vi "RP-GEN SINUS-OUT.vi"(1 "Amplitude(1V)":dbl=1.0, 2 "Frequency (Hz)":i32=2000, 3 "Channel (1|2)":u16(ring)=1 items=["Channel 1"=1, "Channel 2"=2], 4 "IP address":string="192.168.178.107") -> (0 "error out":errorcluster)   [LabVIEW 2021]
uses:
  Red_Pitaya_LabVIEW_Driver&Examples/Red_Pitaya/RedPitaya.lvlib
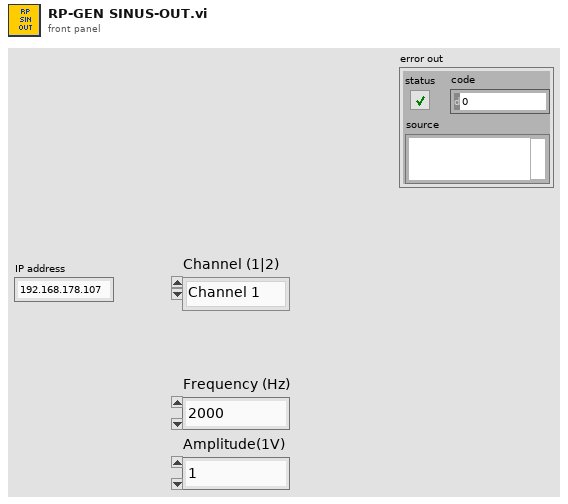
[diagram p1: front panel]
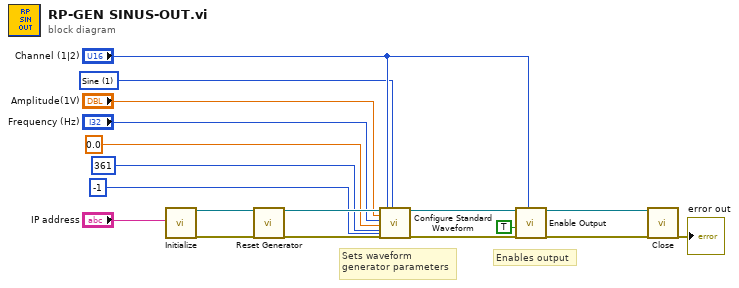
[diagram p0: block diagram]
diagram:
  w6 = u16 1 items=["", "Sine", "Square", "Triangle", "Sawtooth UP", "Sawtooth Down", "PWM"] ("Waveform Function")
  # "Enables output"
  # "Sets waveform\ngenerator parameters"
  n1 = call "Initialize.vi"("IP address"="IP address") -> ("RedPitaya connection out"=w12:refnum<k5>, "error out"=w9:errorcluster)  [unwired: 17 in]
  n2 = call "Reset Generator.vi"("RedPitaya connection in"=w12, "error in"=w9) -> ("RedPitaya connection out"=w11:refnum<k5>, "error out"=w10:errorcluster)  [unwired: 16 in]
  n3 = call "Configure Standard Waveform.vi"("RedPitaya connection in"=w11, "Amplitude (V)"="Amplitude(1V)", "Frequency"="Frequency (Hz)", "DC Offset"=0.0, "Phase"=361, "error in"=w10, "Channel #"="Channel (1|2)", "Duty Cycle"=-1, "Waveform Function"=w6) -> ("RedPitaya connection out"=w16:refnum<k5>, "error out"=w15:errorcluster)  [unwired: 9 in]
  n4 = call "Enable Output.vi"("RedPitaya connection in"=w16, "Generation (T: Enable)"=TRUE, "error in"=w15, "Channel #"="Channel (1|2)") -> ("RedPitaya connection out"=w13:refnum<k5>, "error out"=w14:errorcluster)  [unwired: 14 in]
  n5 = call "Close.vi"("RedPitaya connection in"=w13, "error in"=w14) -> ("error out"=→"error out":errorcluster)  [unwired: 17 in]
